vi "unwrap guid wrapped data.vi"(9 "identifier":string, 10 "uuid":string, 11 "data to unwrap":string) -> (2 "unwrapped data":string, 3 "remaining string":string)   [LabVIEW 2013, in "TBM configuration.lvclass"]
doc: "Parses a dataset of the following form:\n<(additional identifier followed by a space if it is not an empty string)(guid)>(data to unwrap)</(id)(guid)>"
uses:
  TBM configuration.lvclass
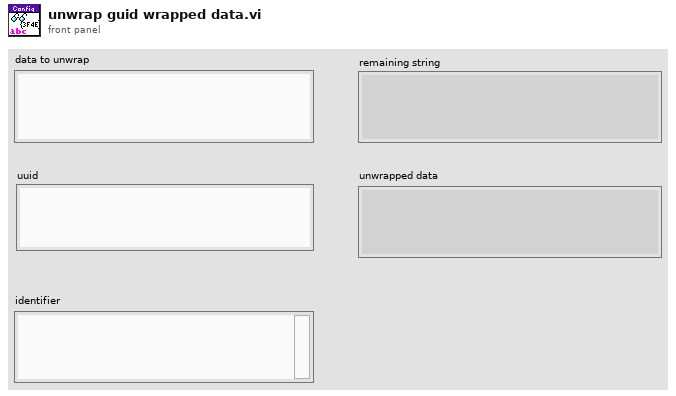
[diagram p1: front panel]
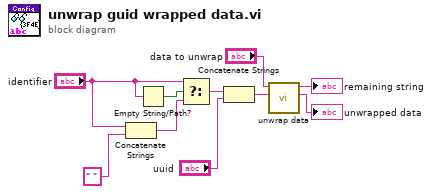
[diagram p0: block diagram]
diagram:
  n1 = Concatenate Strings("identifier", " ") -> (w9:string)
  n2 = Empty String/Path?(string/path="identifier") -> (empty?=w10:bool)
  n3 = Select(t="identifier", s=w10, f=w9) -> (s? t:f=w8:string)
  n4 = Concatenate Strings(w8, "uuid") -> (w2:string)
  n5 = call "unwrap data.vi"("identifier"=w2, "data to unwrap"="data to unwrap") -> ("unwrapped data"=→"unwrapped data":string, "remaining string"=→"remaining string":string)  [unwired: 8 in]
